vi "Get Size of Data from TD - Unknown Type - Returns Error 5000.vi"() -> ()   [LabVIEW 2017, in "Composition.Tests.lvlib"]
uses:
  Composition.Tests.lvlib
  <vilib>/addons/_JKI Toolkits/Caraya/classes/Assert/Assert Error.vi
  Composition/Composition.lvlib
  <vilib>/addons/_JKI Toolkits/Caraya/classes/Assert/Assert.lvclass
  <vilib>/addons/_JKI Toolkits/Caraya/classes/Test/Test.lvclass
panel:
  out "error out":errorcluster
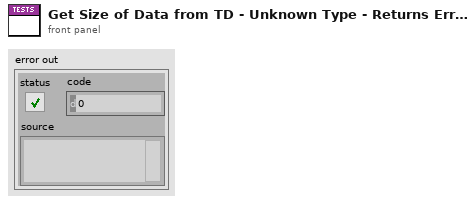
[diagram p1: front panel]
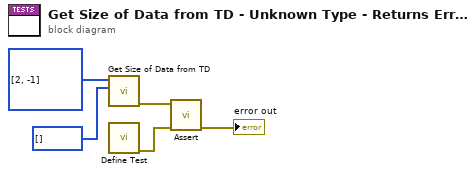
[diagram p0: block diagram]
diagram:
  n1 = call "Get Size of Data from TD.vi"("Data String"=u8[] [], "Type Descriptor"=i16[] [2, -1]) -> ("error out"=w4:errorcluster)  [unwired: 8 in, 1 out]
  n2 = call <vilib>:"Define Test.vi"() -> ("error out"=w3:errorcluster)  [unwired: 11 in]
  n3 = call-poly <vilib>:"Assert.vi"("error in (no error)"=w3, "Error?"=w4) -> ("error out"=→"error out":errorcluster)  [unwired: 9 in]
